vi "BRig_dataCurrent_CueSwitch_Audio.vi"() -> (2 "output_CueSwitch_Audio":i32)   [LabVIEW 2014]
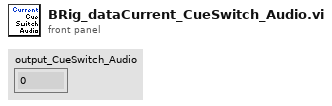
[diagram p1: front panel]
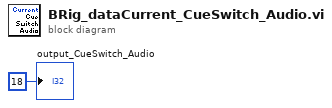
[diagram p0: block diagram]
diagram:
  "output_CueSwitch_Audio" <- 18 ("output_iBlock")
